vi "VI Tree - boolean__ogtk.vi"   [LabVIEW 2009]
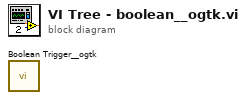
[diagram p0: block diagram]
diagram:
  n1 = call "Boolean Trigger__ogtk.vi"() -> ()  [unwired: 2 in, 2 out]
